vi "Get array index.vi"(0 "Variant in":variant, 5 "brackettedElements":string, 9 "requriedObject":string, 11 "error in (no error)":errorcluster) -> (2 "key":string, 3 "value":string, 4 "indexOut":i32, 6 "Element found?":bool, 8 "Array present?":bool, 10 "VArray":variant, 15 "error out":errorcluster)   [LabVIEW 2015]
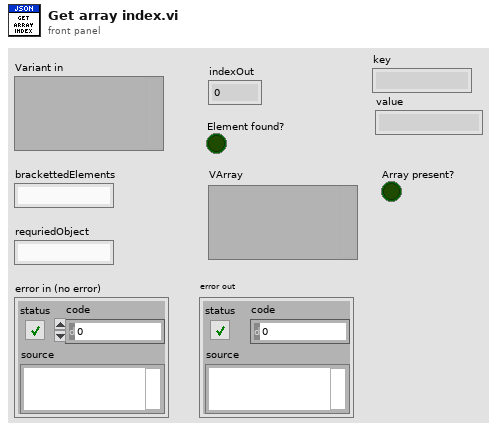
[diagram p1: front panel]
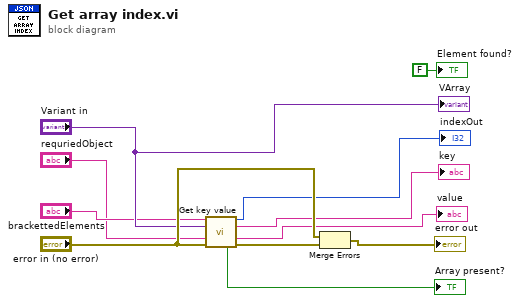
[diagram p0: block diagram]
diagram:
  n1 = call "Get key value.vi"("Single element name"="brackettedElements", "previous\n level\n cluster"="Variant in", "Object name"="requriedObject", "error in (no error)"="error in (no error)") -> ("index out"=→"indexOut":i32, "key"=→"key":string, "value"=→"value":string, "Array Present?"=→"Array present?":bool, "error out"=w11:errorcluster)  [unwired: 5 in, 2 out]
  n2 = Merge Errors("error in (no error)", w11) -> (→"error out":errorcluster)
  "Element found?" <- FALSE ("Element found?")
  "VArray" <- "Variant in"
